vi "VI Shut Down.vi"(8 "Fehler (Eingang, kein Fehler)":errorcluster, 11 "VI Referenz":refnum<vi>) -> (0 "Fehler (Ausgang)":errorcluster, 3 "VI Referenz out":refnum<vi>)   [LabVIEW 2020]
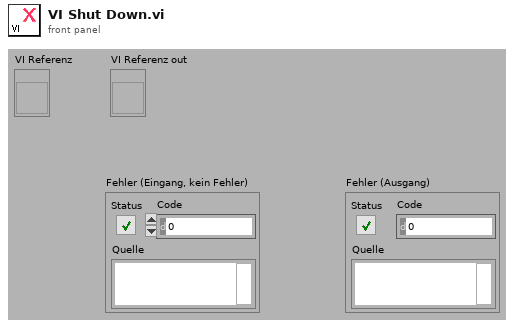
[diagram p1: front panel]
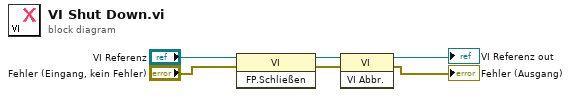
[diagram p0: block diagram]
diagram:
  n1 = invoke class="VI" method="FP.Schließen"(reference="VI Referenz", error in="Fehler (Eingang, kein Fehler)") -> (reference out=w4:refnum<vi>, error out=w3:errorcluster)  [unwired: 1 in, 1 out]
  n2 = invoke class="VI" method="VI Abbr."(reference=w4, error in=w3) -> (error out=→"Fehler (Ausgang)":errorcluster)  [unwired: 1 in, 2 out]
  "VI Referenz out" <- "VI Referenz"
